vi "arduino Motor Control Driver Read Position.vi"(8 "error in (no error)":errorcluster, 10 "Motor ID":u16 max=3 step=1, 11 "Port In":refnum<visa-resource-name>) -> (0 "error out":errorcluster, 1 "Position":i32, 2 "Motor ID dup":u16 max=3 step=1, 3 "Port Out":refnum<visa-resource-name>)   [LabVIEW 2022 SP3]
panel:
  out "Raw Response":string
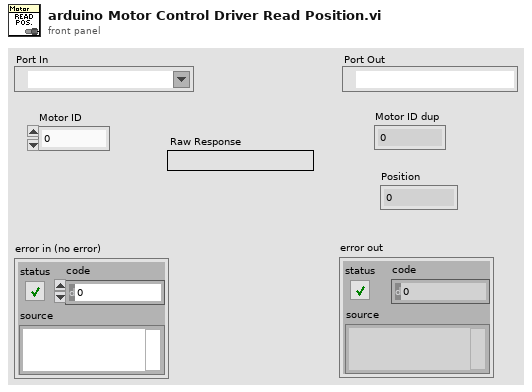
[diagram p1: front panel]
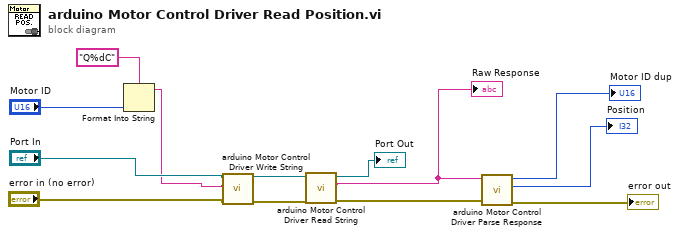
[diagram p0: block diagram]
diagram:
  n1 = Format Into String(format string="Q%dC", "Motor ID") -> (resulting string=w9:string)  [unwired: 2 in, 1 out]
  n2 = call "arduino Motor Control Driver Write String.vi"("error in (no error)"="error in (no error)", "String"=w9, "VISA resource name"="Port In") -> ("error out"=w8:errorcluster, "VISA resource name out"=w7:refnum<visa-resource-name>)  [unwired: 7 in]
  n3 = call "arduino Motor Control Driver Read String.vi"("error in (no error)"=w8, "reference"=w7) -> ("error out"=w2:errorcluster, "response"=w6:string, "reference out"=→"Port Out":refnum<visa-resource-name>)  [unwired: 7 in]
  "Raw Response" <- w6
  n4 = call "arduino Motor Control Driver Parse Response.vi"("error in"=w2, "Q cmd response"=w6) -> ("error out"=→"error out":errorcluster, "pos"=→"Position":i32, "m"=→"Motor ID dup":i32)  [unwired: 7 in]
